vi "PSVCH_Refresh VCH Formula.vi"(8 "error in":errorcluster, 9 "Formula In":string, 10 "String":string, 11 "VCH_Formula":refnum<vi>) -> (0 "error out":errorcluster, 2 "result string":string)   [LabVIEW 2016]
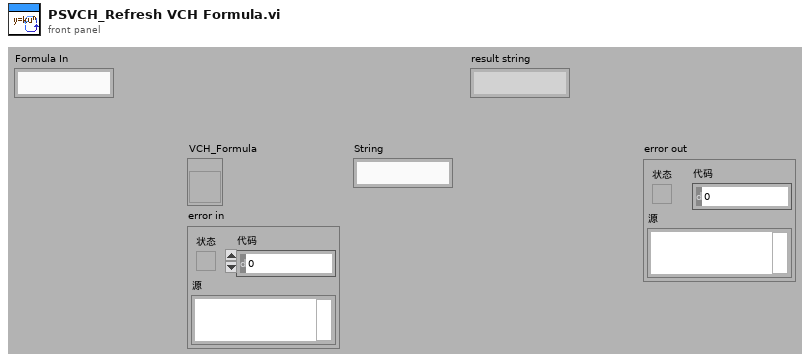
[diagram p1: front panel]
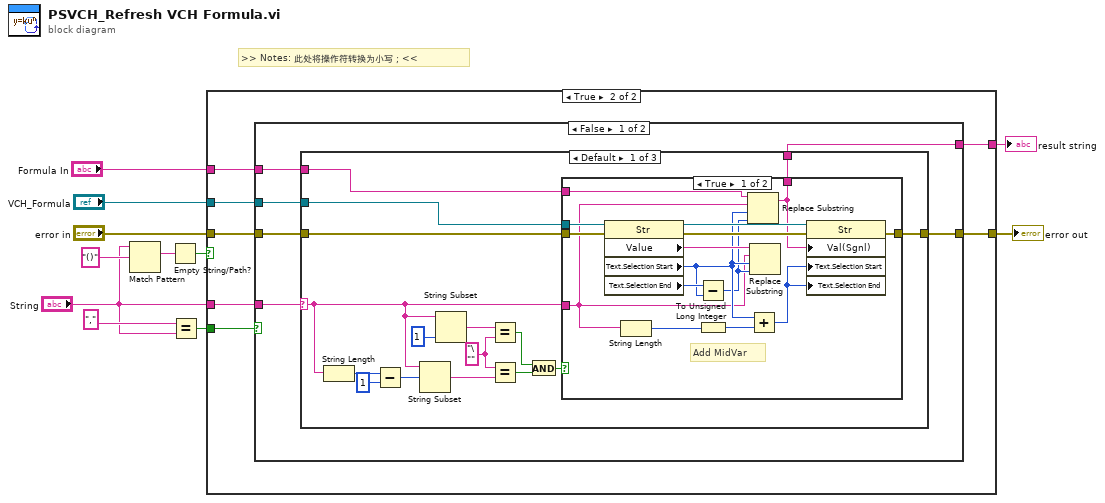
[diagram p0: block diagram]
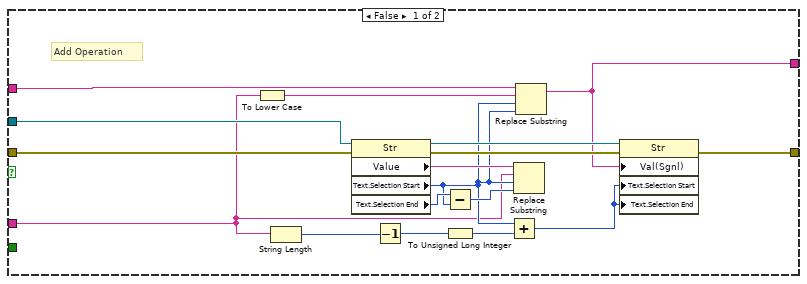
[diagram p2: hidden frame]
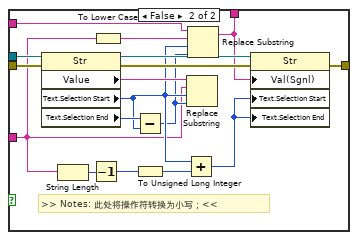
[diagram p3: hidden frame]
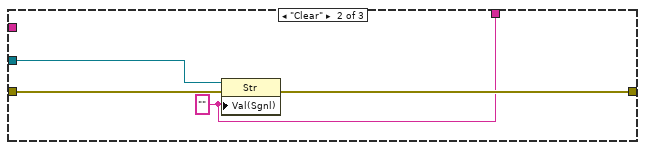
[diagram p4: hidden frame]
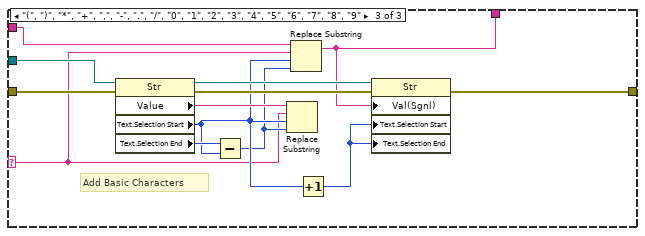
[diagram p5: hidden frame]
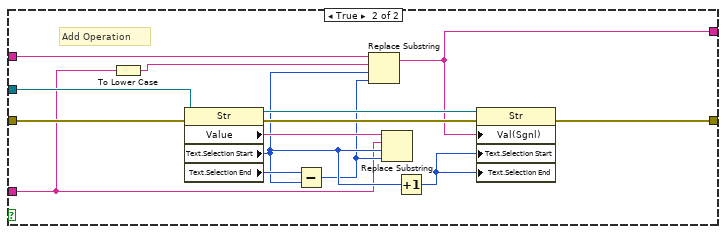
[diagram p6: hidden frame]
diagram:
  # ">> Notes: 此处将操作符转换为小写；<<"
  n1 = Match Pattern(string="String", regular expression="()" ("正则表达式")) -> (match substring=w6:string)  [unwired: 1 in, 3 out]
  n2 = Empty String/Path?(string/path=w6) -> (empty?=w3:bool)
  n3 = Equal?(x=",", y="String") -> (x = y?=w10:bool)
  n4 = case shown="True" w3 {
    tunnel: w10 -> [_ w35]
    tunnel: "VCH_Formula" -> [w18 w34]
    tunnel: [w17 w33] -> w8
    tunnel: "error in" -> [w19 w32]
    tunnel: "String" -> [w14 w31]
    tunnel: [w12 w30] -> w2
    tunnel: "Formula In" -> [w16 w29]
    frame False {
      # "Add Operation"
      n5 = To Lower Case(string=w14) -> (all lower case string=w13:string)
      n6 = String Length(string=w14) -> (length=w22:i32)
      n7 = property class="Str"(reference=w18, error in=w19) -> (reference out=w24:refnum<vi>, error out=w25:errorcluster, "Value"=w27:string, "Text.Selection Start"=w15:u32, "Text.Selection End"=w28:u32)
      n8 = Decrement(x=w22) -> (x-1=w21:i32)
      n9 = Subtract(x=w28, y=w15) -> (x-y=w26:u32)
      n10 = To Unsigned Long Integer(number=w21) -> (unsigned 32bit integer=w20:u32)
      n11 = Add(x=w15, y=w20) -> (x+y=w23:u32)
      n12 = Replace Substring(2:w26, 3:w15, 4:w14, 5:w27) -> ()  [unwired: 2 out]
      n13 = Replace Substring(2:w15, 3:w15, 4:w13, 5:w16) -> (1:w12:string)  [unwired: 1 out]
      n14 = property class="Str"(reference=w24, error in=w25, "Val(Sgnl)"=w12, "Text.Selection Start"=w23, "Text.Selection End"=w23) -> (error out=w17:errorcluster)  [unwired: 1 out]
    }
    frame True {
      n15 = case shown="False" w35 {
        tunnel: w32 -> [w41 w115]
        tunnel: w34 -> [w40 w114]
        tunnel: w31 -> [w39 w109]
        tunnel: [w38 w113] -> w33
        tunnel: [w37 w107] -> w30
        tunnel: w29 -> [w36 w112]
        frame False {
          n16 = case shown="Default" w39 {
            selector: w39 -> [w45 _ w95]
            tunnel: w41 -> [w47 w93 w106]
            tunnel: w40 -> [w46 w92 w105]
            tunnel: [w44 w91 w100] -> w38
            tunnel: [w43 w90 w94] -> w37
            tunnel: w36 -> [w42 _ w98]
            frame Default {
              w51 = "\""
              n17 = String Length(string=w45) -> (length=w56:i32)
              n18 = Subtract(x=w56, y=1) -> (x-y=w55:i32)
              n19 = String Subset(string=w45, offset (0)=w55) -> (substring=w53:string)  [unwired: 1 in]
              n20 = String Subset(string=w45, length (rest)=1 ("length (rest)")) -> (substring=w52:string)  [unwired: 1 in]
              n21 = Equal?(x=w52, y=w51) -> (x = y?=w50:bool)
              n22 = Equal?(x=w51, y=w53) -> (x = y?=w49:bool)
              n23 = And(x=w50, y=w49) -> (x .and. y?=w48:bool)
              n24 = case shown="True" w48 {
                tunnel: w47 -> [w66 w83]
                tunnel: w46 -> [w65 w82]
                tunnel: w45 -> [w59 w75]
                tunnel: [w63 w80] -> w44
                tunnel: [w58 w73] -> w43
                tunnel: w42 -> [w62 w78]
                frame True {
                  # "Add MidVar"
                  n25 = property class="Str"(reference=w65, error in=w66) -> (reference out=w70:refnum<vi>, error out=w69:errorcluster, "Value"=w68:string, "Text.Selection Start"=w61:u32, "Text.Selection End"=w67:u32)
                  n26 = String Length(string=w59) -> (length=w64:i32)
                  n27 = Subtract(x=w67, y=w61) -> (x-y=w60:u32)
                  n28 = To Unsigned Long Integer(number=w64) -> (unsigned 32bit integer=w72:u32)
                  n29 = Replace Substring(2:w60, 3:w61, 4:w59, 5:w62) -> (1:w58:string)  [unwired: 1 out]
                  n30 = Add(x=w61, y=w72) -> (x+y=w71:u32)
                  n31 = Replace Substring(2:w60, 3:w61, 4:w59, 5:w68) -> ()  [unwired: 2 out]
                  n32 = property class="Str"(reference=w70, error in=w69, "Val(Sgnl)"=w58, "Text.Selection Start"=w71, "Text.Selection End"=w71) -> (error out=w63:errorcluster)  [unwired: 1 out]
                }
                frame False {
                  # ">> Notes: 此处将操作符转换为小写；<<"
                  n33 = property class="Str"(reference=w82, error in=w83) -> (reference out=w87:refnum<vi>, error out=w86:errorcluster, "Value"=w85:string, "Text.Selection Start"=w77:u32, "Text.Selection End"=w84:u32)
                  n34 = String Length(string=w75) -> (length=w81:i32)
                  n35 = Decrement(x=w81) -> (x-1=w79:i32)
                  n36 = To Lower Case(string=w75) -> (all lower case string=w74:string)
                  n37 = Subtract(x=w84, y=w77) -> (x-y=w76:u32)
                  n38 = To Unsigned Long Integer(number=w79) -> (unsigned 32bit integer=w89:u32)
                  n39 = Add(x=w77, y=w89) -> (x+y=w88:u32)
                  n40 = Replace Substring(2:w76, 3:w77, 4:w75, 5:w85) -> ()  [unwired: 2 out]
                  n41 = Replace Substring(2:w76, 3:w77, 4:w74, 5:w78) -> (1:w73:string)  [unwired: 1 out]
                  n42 = property class="Str"(reference=w87, error in=w86, "Val(Sgnl)"=w73, "Text.Selection Start"=w88, "Text.Selection End"=w88) -> (error out=w80:errorcluster)  [unwired: 1 out]
                }
              }
            }
            frame "Clear" {
              w90 = "" ("Value")
              n43 = property class="Str"(reference=w92, error in=w93, "Val(Sgnl)"=w90) -> (error out=w91:errorcluster)  [unwired: 1 out]
            }
            frame "(", ")", "*", "+", ",", "-", ".", "/", "0", "1", "2", "3", "4", "5", "6", "7", "8", "9" {
              # "Add Basic Characters"
              n44 = property class="Str"(reference=w105, error in=w106) -> (reference out=w101:refnum<vi>, error out=w102:errorcluster, "Value"=w103:string, "Text.Selection Start"=w97:u32, "Text.Selection End"=w104:u32)
              n45 = Subtract(x=w104, y=w97) -> (x-y=w96:u32)
              n46 = Replace Substring(2:w96, 3:w97, 4:w95, 5:w103) -> ()  [unwired: 2 out]
              n47 = Replace Substring(2:w96, 3:w97, 4:w95, 5:w98) -> (1:w94:string)  [unwired: 1 out]
              n48 = Increment(x=w97) -> (x+1=w99:u32)
              n49 = property class="Str"(reference=w101, error in=w102, "Val(Sgnl)"=w94, "Text.Selection Start"=w99, "Text.Selection End"=w99) -> (error out=w100:errorcluster)  [unwired: 1 out]
            }
          }
        }
        frame True {
          # "Add Operation"
          n50 = To Lower Case(string=w109) -> (all lower case string=w108:string)
          n51 = property class="Str"(reference=w114, error in=w115) -> (reference out=w117:refnum<vi>, error out=w118:errorcluster, "Value"=w119:string, "Text.Selection Start"=w111:u32, "Text.Selection End"=w120:u32)
          n52 = Subtract(x=w120, y=w111) -> (x-y=w110:u32)
          n53 = Replace Substring(2:w110, 3:w111, 4:w108, 5:w112) -> (1:w107:string)  [unwired: 1 out]
          n54 = Replace Substring(2:w110, 3:w111, 4:w109, 5:w119) -> ()  [unwired: 2 out]
          n55 = Increment(x=w111) -> (x+1=w116:u32)
          n56 = property class="Str"(reference=w117, error in=w118, "Val(Sgnl)"=w107, "Text.Selection Start"=w116, "Text.Selection End"=w116) -> (error out=w113:errorcluster)  [unwired: 1 out]
        }
      }
    }
  }
  "error out" <- w8
  "result string" <- w2
